vi "Main.vi"() -> ()   [LabVIEW 2011]
uses:
  granula_llb.lvlib
panel:
  out "tdms path":string caption="ЗАДАНИЕ, мин"
  in  "Участок 2 выключить":bool
  out "Проведение второго участка":bool
  in  "участок 2 включить":bool
  in  "Cal v 2":i16
  in  "S2 t 2":i16
  in  "S2v 2":i16
  in  "S1 t 2":i16
  in  "S1 v 2":i16
  in  "МАКРО СТОП":bool
  in  "НАГРЕВ НАЧАТЬ АВТО":bool
  in  "ВЫГРУЗИТЬ":bool
  in  "ЗАГРУЗИТЬ":bool
  out "T7":string caption="Т7"
  in  "Cal v":i16
  in  "S2 t":i16
  in  "S2v":i16
  in  "S1 t":i16
  in  "S1 v":i16
  in  "A":i16
  in  "Hz":i16
  in  "T7":i16
  in  "T6":i16
  in  "T5":i16
  in  "T4":i16
  in  "T3":i16
  in  "T2":i16
  in  "T1":i16
  in  "error":i16
  out "Нагрев включен":bool caption="Нагрев"
  out "Готовность привода":bool caption="Готов"
  out "Авария привода":bool caption="Авария"
  in  "Y20-Y57":i32
  in  "X100-X137":i32
  in  "X40-X77":i32
  out "Команда выход":bool caption="ОТКРЫТ"
  in  "Закалка выкл":bool
  in  "Закалка вкл":bool
  in  "Телегу в точку А":bool
  in  "Телегу под печь":bool
  in  "Телегу на разгрузку":bool
  in  "Под закрыть":bool
  in  "ПОД открыnnть":bool
  in  "Цепи вниз":bool
  in  "Цепи наверх":bool
  in  "Домкрат вверх":bool
  in  "Домкрат вниз":bool
  out "Закалка":bool
  out "Участок 2":bool
  out "Участок 1":bool
  out "АВТО ЦИКЛ":bool
  out "текущее время":string
  in  "Цикл пуск":bool
  in  "Цикл стоп":bool
  in  "Просмотр графика":bool
  in  "Наладка":bool
  in  "ВЫХОД":bool
  out "УПРАВЛЕНИЕ С PLC":bool
  out "ВОДА":bool
  out "ВОДА 2":bool
  out "ВОДА 3":bool
  out "ВОДА 4":bool
  out "Проведение закалки":bool
  out "Зак зад":string caption="ЗАДАНИЕ, мин"
  out "Зак выд":string caption="ВЫДЕРЖКА, мин"
  out "Уч2 Тзад":string caption="ЗАДАНИЕ, град"
  out "Уч2 Т":string caption="ТЕМПЕРАТУРА, град"
  out "Уч2 Выд зад":string caption="ЗАДАНИЕ, мин"
  out "Уч2 Выд":string caption="ВЫДЕРЖКА, мин"
  out "Уч1 Т зад":string caption="ЗАДАНИЕ, град"
  out "Уч1 Т":string caption="ТЕМПЕРАТУРА, град"
  out "Уч1 выд зад":string caption="ЗАДАНИЕ, мин"
  out "Уч1 Выд":string caption="ВЫДЕРЖКА, мин"
  out "ПОД ЗАКРЫТ":bool caption="ЗАКРЫТ"
  out "ПОД ОТКРЫТ":bool caption="ОТКРЫТ"
  out "Двиг Ток А":string caption="ТОК А"
  out "Двиг част Hz":string caption="ЧАСТОТА Hz"
  out "T5":string caption="Т5"
  out "T6":string caption="Т6"
  out "T3":string caption="Т3"
  out "T4":string caption="Т4"
  out "T1":string caption="Т1"
  out "T2":string caption="Т2"
  out "ТОЧКА А":bool
  out "ЗАЦЕП":bool
  out "РАЗГРУЗКА":bool
  out "Цепи внизу":bool caption="Закал"
  out "Цепи среднее":bool caption="Зацеп"
  out "Цепи вверху":bool caption="Камера"
  out "Домкрат внизу":bool caption="Закал"
  out "Домкрат вверху":bool caption="Зацеп"
  # "КАМЕРА НАГРЕВА"
  # "НАГРЕВ"
  # "МАКРО"
  # "ПОД"
  # "ЦЕПИ"
  # "Д\nО\nМ\nК\nР\nА\nТ"
  # "Д\nО\nМ\nК\nР\nА\nТ"
  # "САДКА"
  # "Т\nЕ\nЛ\nЕ\nГ\nА"
  # "САДКА"
  # "ИНДИКАЦИЯ ПРОТОКА ВОДЫ"
  # "СТУПЕНЬ №2"
  # "СТУПЕНЬ №1"
  # "ЗАКАЛКА"
  # "ПРОВЕДЕНИЕ ЗАКАЛКИ"
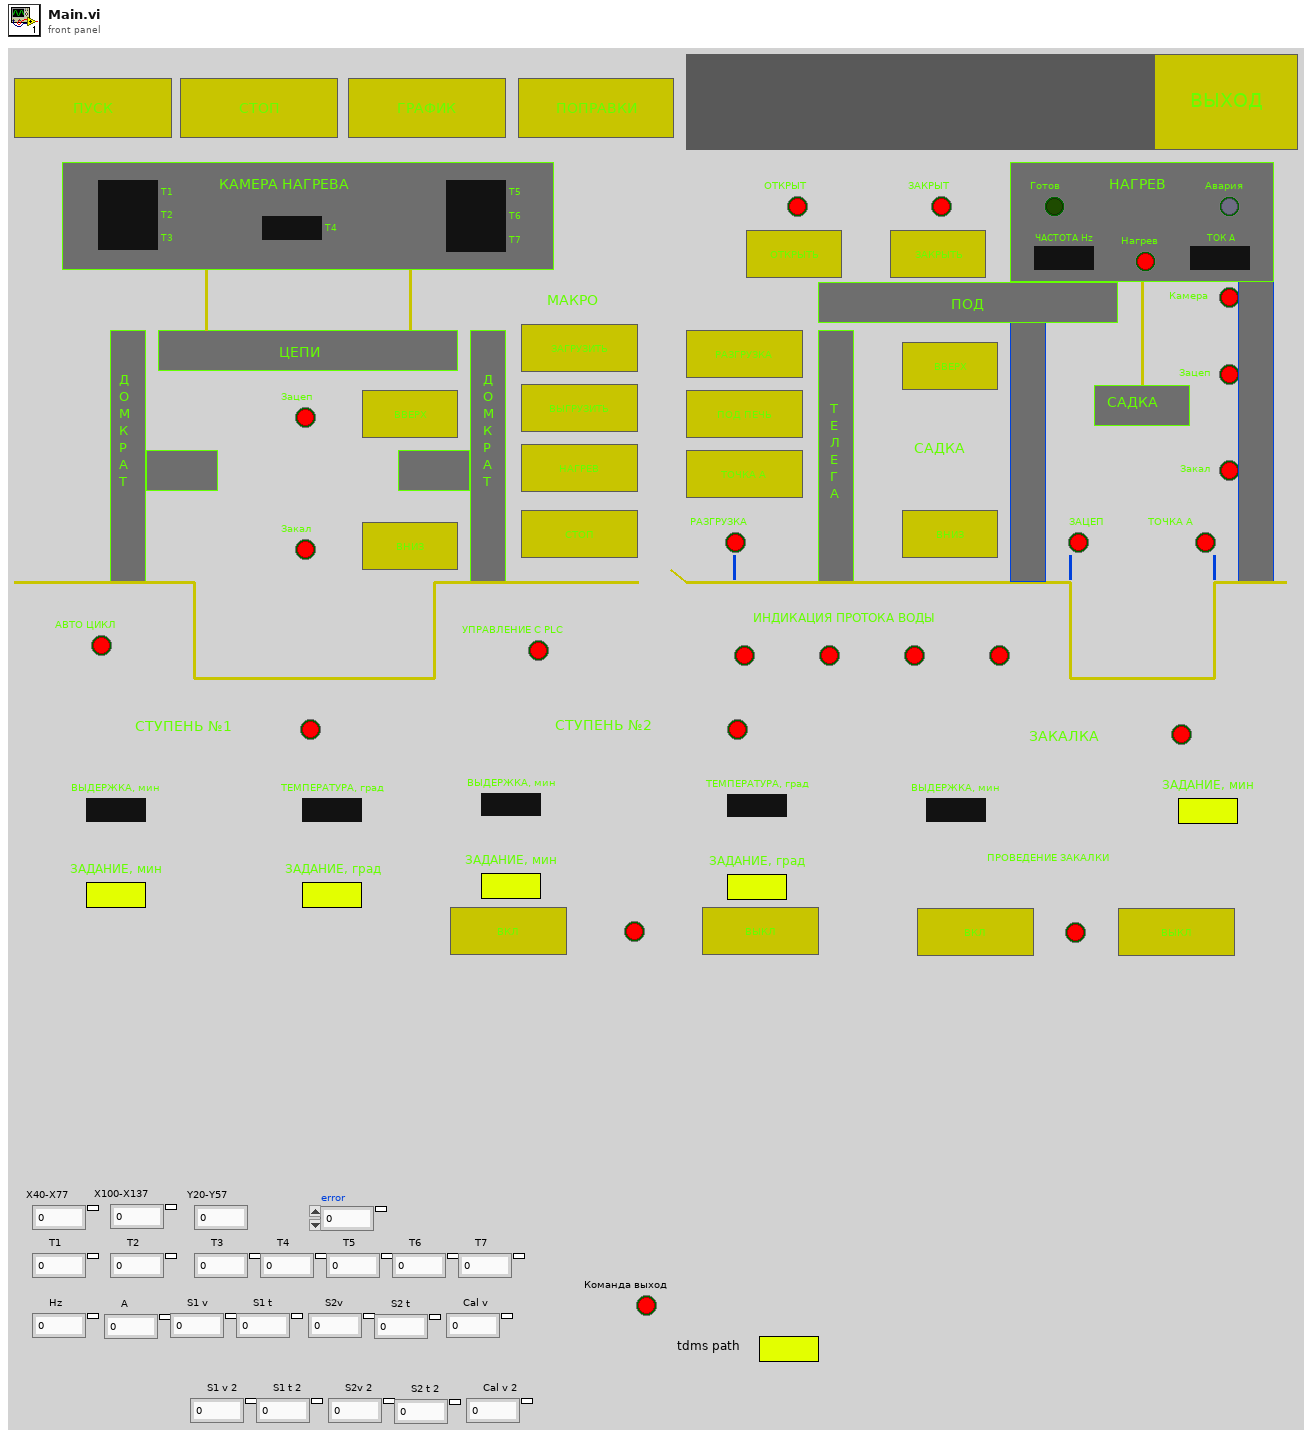
[diagram p1: front panel]
types:
  T1 = enum16{"big-endian, network order", "native, host order", "little-endian"}
  T2 = enum16{"open", "open or create", "create or replace", "create", "open (read-only)"}
  T3 = enum16{"open", "replace", "create", "open or create", "replace or create", "replace or create with confirmation"}
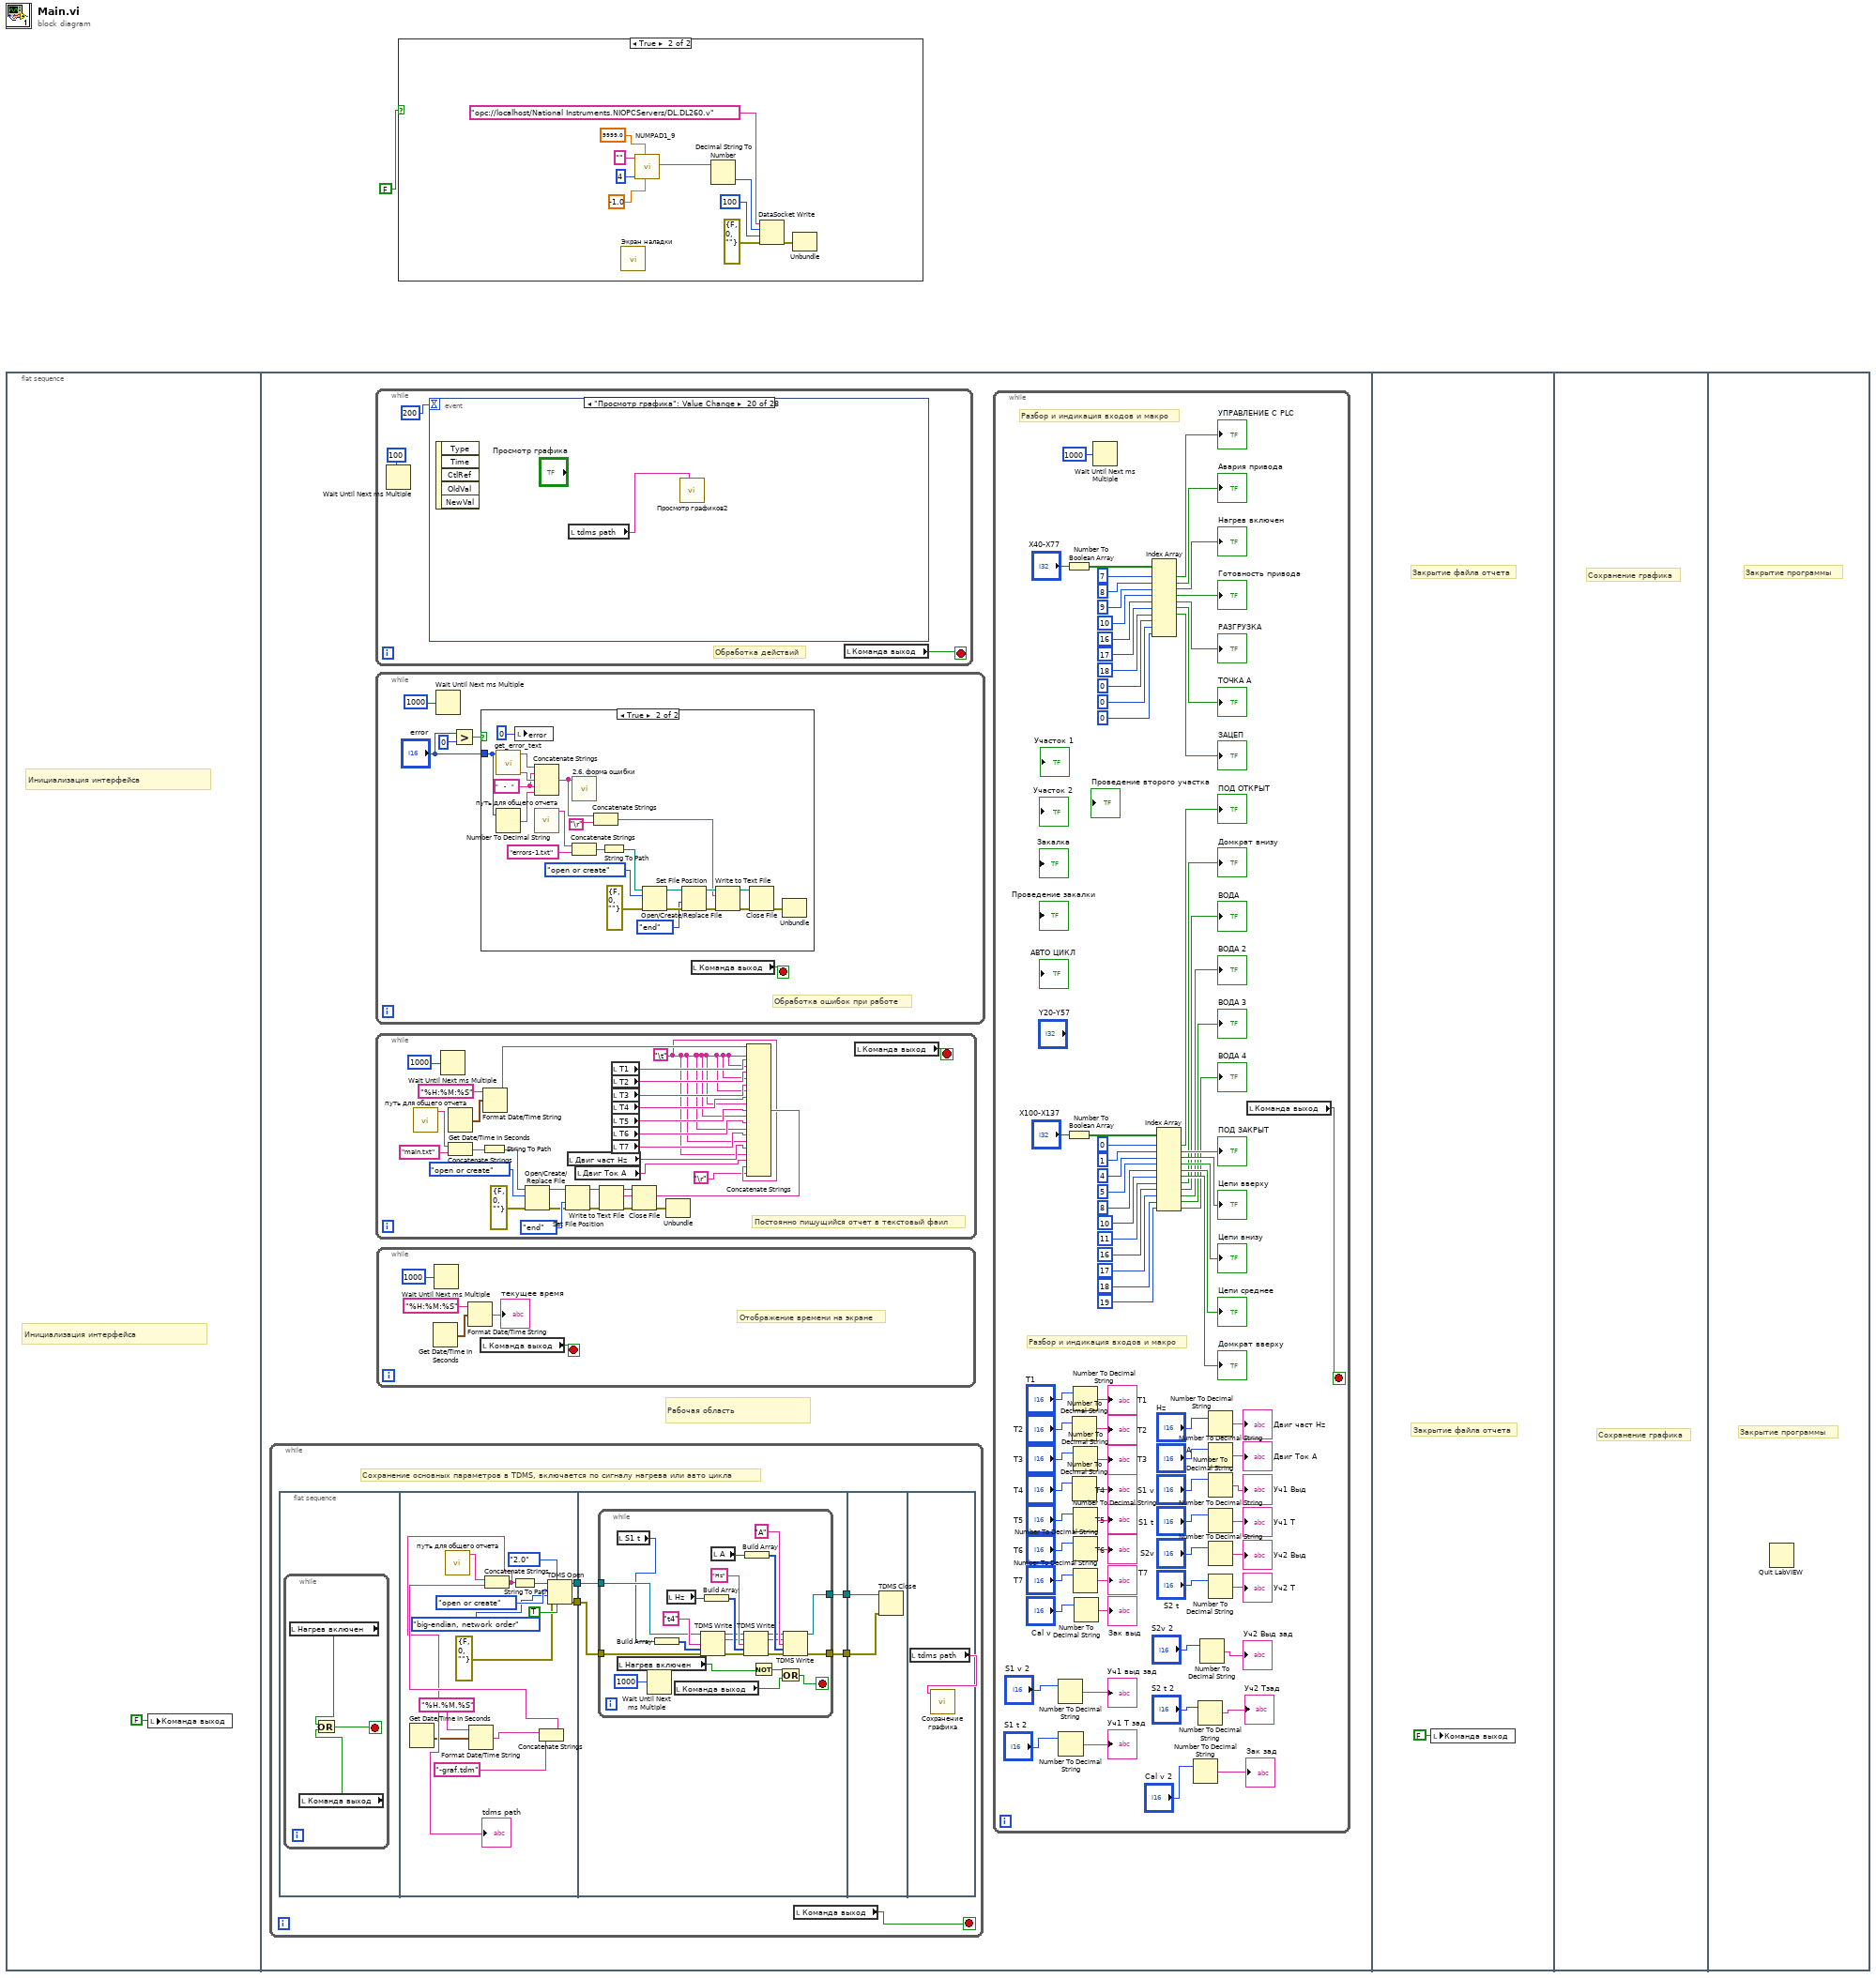
[diagram p0: block diagram]
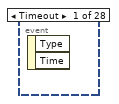
[diagram p3: hidden frame]
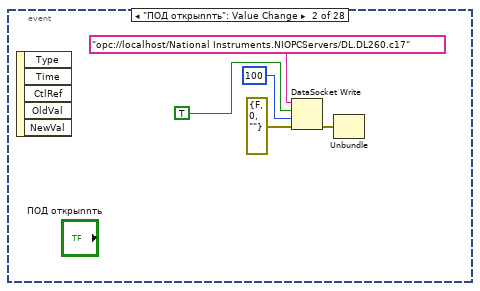
[diagram p4: hidden frame]
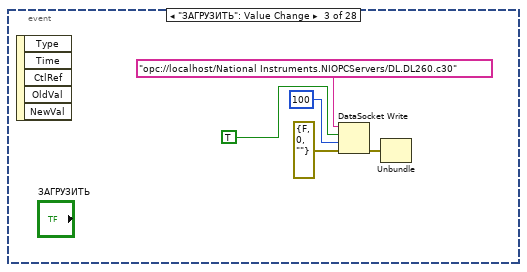
[diagram p5: hidden frame]
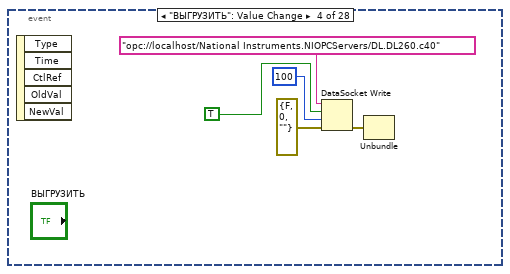
[diagram p6: hidden frame]
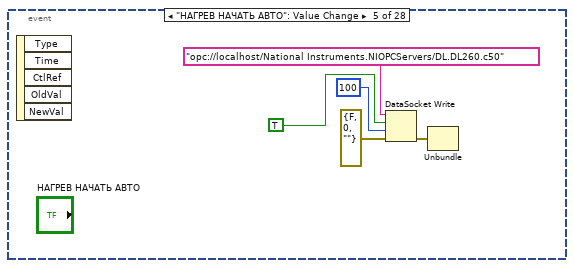
[diagram p7: hidden frame]
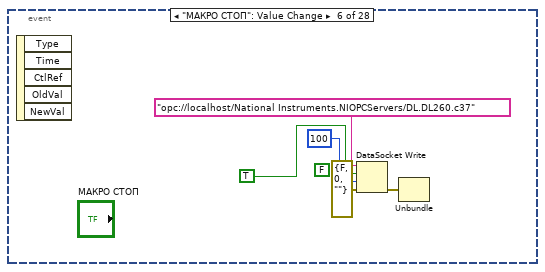
[diagram p8: hidden frame]
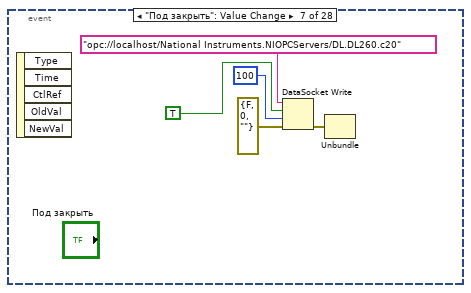
[diagram p9: hidden frame]
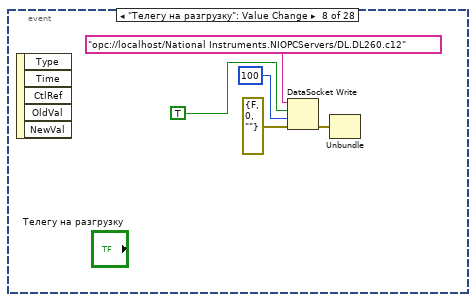
[diagram p10: hidden frame]
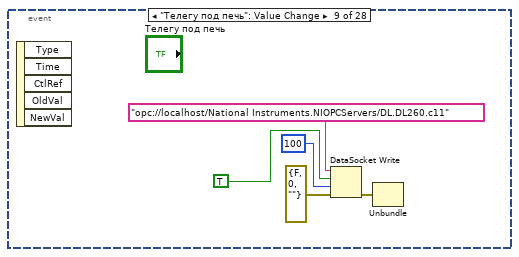
[diagram p11: hidden frame]
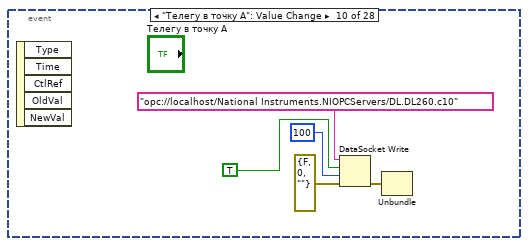
[diagram p12: hidden frame]
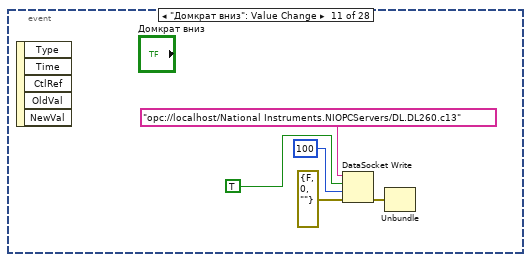
[diagram p13: hidden frame]
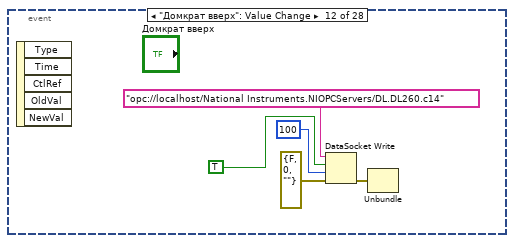
[diagram p14: hidden frame]
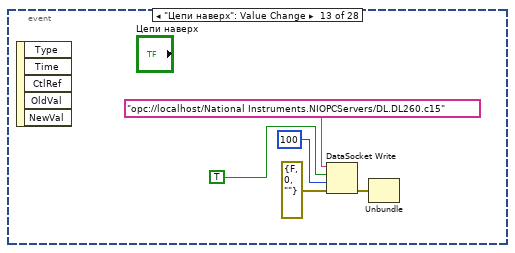
[diagram p15: hidden frame]
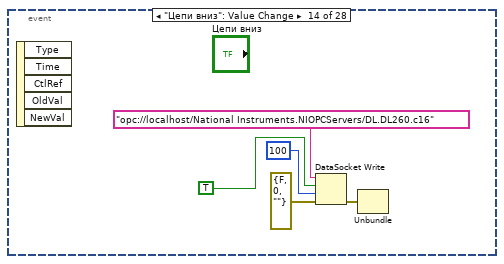
[diagram p16: hidden frame]
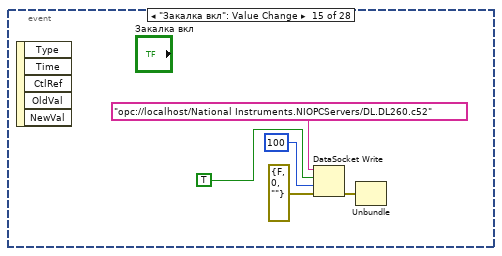
[diagram p17: hidden frame]
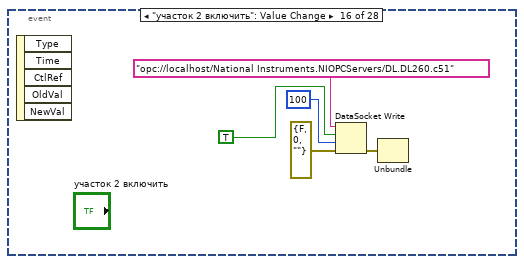
[diagram p18: hidden frame]
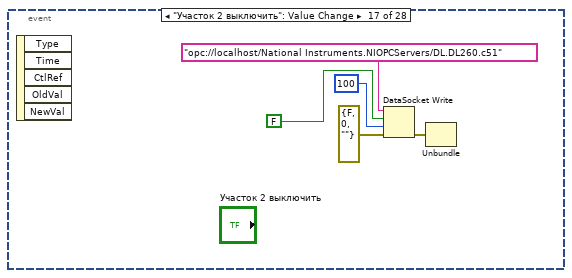
[diagram p19: hidden frame]
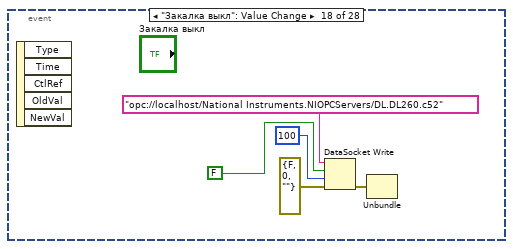
[diagram p20: hidden frame]
diagram:
  n1 = flat-sequence {
    frame #0 {
      # "Инициализация интерфейса"
      # "Инициализация интерфейса"
      n2 = local write "Команда выход"(FALSE ("Команда выход")) -> ()
    }
    frame #1 {
      # "Рабочая область"
      n3 = while {
        stop <- w3 stop-if-true
        # "Сохранение основных параметров в TDMS, включается по сигналу нагрева или авто цикла"
        n4 = flat-sequence {
          tunnel: [w16] -> w7
          tunnel: [w15] -> w6
          tunnel: w7 -> [w29]
          tunnel: w6 -> [w28]
          tunnel: [w27] -> w5
          tunnel: [w26] -> w4
          tunnel: w5 -> [w55]
          tunnel: w4 -> [w54]
          frame #0 {
            n5 = while {
              stop <- w10 stop-if-true
              n6 = local read "Нагрев включен"() -> (w8:bool)
              n7 = local read "Команда выход"() -> (w9:bool)
              n8 = Or(x=w8, y=w9) -> (x .or. y?=w10:bool)
            }
          }
          frame #1 {
            n9 = Get Date/Time In Seconds() -> (seconds since 1Jan1904=w11:timestamp)
            n10 = call "путь для общего отчета.vi"() -> ("path_out 2"=w25:string)  [unwired: 11 in]
            n11 = Format Date/Time String(time format string (%c)="%H.%M.%S", seconds (now)=w11) -> (date/time string=w13:string)  [unwired: 1 in]
            n12 = Concatenate Strings(w13, "-graf.tdm") -> (w17:string)
            n13 = Concatenate Strings(w25, w17) -> (w14:string)
            "tdms path" <- w14
            n14 = String To Path(string=w14) -> (path=w24:path)
            n15 = TDMS Open(6:TRUE ("disable buffering? (T)"), 7:enum16{"1.0", "2.0"}."2.0" ("file format version (2.0)"), 8:errorcluster {"status"=FALSE, "code"=0, "source"=""} ("error in (no error)"), 9:T1."big-endian, network order" ("byte order (2:little-endian)"), 10:T2."open or create" ("operation (0:open)"), 11:w24) -> (0:w15:errorcluster, 3:w16:refnum<k34>)
          }
          frame #2 {
            n16 = while {
              tunnel: w29 -> [w38]
              tunnel: w28 -> [w37]
              tunnel: [w36] -> w27
              tunnel: [w35] -> w26
              stop <- w32 stop-if-true
              n17 = local read "S1 t"() -> (w30:i16)
              n18 = local read "Нагрев включен"() -> (w31:bool)
              n19 = Wait Until Next ms Multiple(millisecond multiple=u32 1000) -> ()  [unwired: 1 out]
              n20 = Build Array(w30) -> (w53:i16[])
              n21 = local read "Hz"() -> (w44:i16)
              n22 = local read "Команда выход"() -> (w33:bool)
              n23 = TDMS Write(0:w38, 7:"t4", 9:w53, 11:w37) -> (4:w42:refnum<k34>, 6:w41:string, 15:w40:errorcluster)  [unwired: 2 in, 1 out]
              n24 = Build Array(w44) -> (w50:i16[])
              n25 = local read "A"() -> (w45:i16)
              n26 = TDMS Write(0:w42, 5:w41, 7:"Hz", 9:w50, 11:w40) -> (4:w47:refnum<k34>, 6:w43:string, 15:w46:errorcluster)  [unwired: 1 in, 1 out]
              n27 = Build Array(w45) -> (w48:i16[])
              n28 = Not(x=w31) -> (.not. x?=w34:bool)
              n29 = Or(x=w34, y=w33) -> (x .or. y?=w32:bool)
              n30 = TDMS Write(0:w47, 5:w43, 7:"A", 9:w48, 11:w46) -> (4:w36:refnum<k34>, 15:w35:errorcluster)  [unwired: 1 in, 2 out]
            }
          }
          frame #3 {
            n31 = TDMS Close(8:w54, 11:w55) -> ()  [unwired: 2 out]
          }
          frame #4 {
            n32 = local read "tdms path"() -> (w56:string)
            n33 = call "Сохранение графика.vi"("String"=w56) -> ()  [unwired: 11 in]
          }
        }
        n34 = local read "Команда выход"() -> (w3:bool)
      }
      n35 = while {
        stop <- w62 stop-if-true
        # "Обработка действий"
        n36 = Wait Until Next ms Multiple(millisecond multiple=u32 100) -> ()  [unwired: 1 out]
        n37 = event shown="[19] \"Просмотр графика\": Value Change" {
          selector: _ -> [_ _ _ _ _ _ _ _ _ _ _ _ _ _ _ _ _ _ _ _ _ _ _ _ _ _ _ _]
          dyn-events: _ -> [_ _ _ _ _ _ _ _ _ _ _ _ _ _ _ _ _ _ _ _ _ _ _ _ _ _ _ _]
          timeout: 200 -> [_ _ _ _ _ _ _ _ _ _ _ _ _ _ _ _ _ _ _ _ _ _ _ _ _ _ _ _]
          event Timeout {
            n38 = event-data() -> ()  [unwired: 1 in, 2 out]
          }
          event "ПОД открыnnть": Value Change {
            n39 = event-data() -> ()  [unwired: 1 in, 5 out]
            n40 = DataSocket Write(8:errorcluster {"status"=FALSE, "code"=0, "source"=""} ("error in (no error)"), 9:100 ("ms timeout (0)"), 10:TRUE, 11:"opc://localhost/National Instruments.NIOPCServers/DL.DL260.c17" ("connection in")) -> (0:w69:errorcluster)  [unwired: 2 out]
            n41 = Unbundle(w69) -> ()  [unwired: 3 out]
          }
          event "ЗАГРУЗИТЬ": Value Change {
            n42 = event-data() -> ()  [unwired: 1 in, 5 out]
            n43 = DataSocket Write(8:errorcluster {"status"=FALSE, "code"=0, "source"=""} ("error in (no error)"), 9:100 ("ms timeout (0)"), 10:TRUE, 11:"opc://localhost/National Instruments.NIOPCServers/DL.DL260.c30" ("connection in")) -> (0:w74:errorcluster)  [unwired: 2 out]
            n44 = Unbundle(w74) -> ()  [unwired: 3 out]
          }
          event "ВЫГРУЗИТЬ": Value Change {
            n45 = event-data() -> ()  [unwired: 1 in, 5 out]
            n46 = DataSocket Write(8:errorcluster {"status"=FALSE, "code"=0, "source"=""} ("error in (no error)"), 9:100 ("ms timeout (0)"), 10:TRUE, 11:"opc://localhost/National Instruments.NIOPCServers/DL.DL260.c40" ("connection in")) -> (0:w79:errorcluster)  [unwired: 2 out]
            n47 = Unbundle(w79) -> ()  [unwired: 3 out]
          }
          event "НАГРЕВ НАЧАТЬ АВТО": Value Change {
            n48 = event-data() -> ()  [unwired: 1 in, 5 out]
            n49 = DataSocket Write(8:errorcluster {"status"=FALSE, "code"=0, "source"=""} ("error in (no error)"), 9:100 ("ms timeout (0)"), 10:TRUE, 11:"opc://localhost/National Instruments.NIOPCServers/DL.DL260.c50" ("connection in")) -> (0:w84:errorcluster)  [unwired: 2 out]
            n50 = Unbundle(w84) -> ()  [unwired: 3 out]
          }
          event "МАКРО СТОП": Value Change {
            (unwired) FALSE ("status")
            n51 = event-data() -> ()  [unwired: 1 in, 5 out]
            n52 = DataSocket Write(8:errorcluster {"status"=FALSE, "code"=0, "source"=""} ("error in (no error)"), 9:100 ("ms timeout (0)"), 10:TRUE, 11:"opc://localhost/National Instruments.NIOPCServers/DL.DL260.c37" ("connection in")) -> (0:w89:errorcluster)  [unwired: 2 out]
            n53 = Unbundle(w89) -> ()  [unwired: 3 out]
          }
          event "Под закрыть": Value Change {
            n54 = event-data() -> ()  [unwired: 1 in, 5 out]
            n55 = DataSocket Write(8:errorcluster {"status"=FALSE, "code"=0, "source"=""} ("error in (no error)"), 9:100 ("ms timeout (0)"), 10:TRUE, 11:"opc://localhost/National Instruments.NIOPCServers/DL.DL260.c20" ("connection in")) -> (0:w94:errorcluster)  [unwired: 2 out]
            n56 = Unbundle(w94) -> ()  [unwired: 3 out]
          }
          event "Телегу на разгрузку": Value Change {
            n57 = event-data() -> ()  [unwired: 1 in, 5 out]
            n58 = DataSocket Write(8:errorcluster {"status"=FALSE, "code"=0, "source"=""} ("error in (no error)"), 9:100 ("ms timeout (0)"), 10:TRUE, 11:"opc://localhost/National Instruments.NIOPCServers/DL.DL260.c12" ("connection in")) -> (0:w99:errorcluster)  [unwired: 2 out]
            n59 = Unbundle(w99) -> ()  [unwired: 3 out]
          }
          event "Телегу под печь": Value Change {
            n60 = event-data() -> ()  [unwired: 1 in, 5 out]
            n61 = DataSocket Write(8:errorcluster {"status"=FALSE, "code"=0, "source"=""} ("error in (no error)"), 9:100 ("ms timeout (0)"), 10:TRUE, 11:"opc://localhost/National Instruments.NIOPCServers/DL.DL260.c11" ("connection in")) -> (0:w104:errorcluster)  [unwired: 2 out]
            n62 = Unbundle(w104) -> ()  [unwired: 3 out]
          }
          event "Телегу в точку А": Value Change {
            n63 = event-data() -> ()  [unwired: 1 in, 5 out]
            n64 = DataSocket Write(8:errorcluster {"status"=FALSE, "code"=0, "source"=""} ("error in (no error)"), 9:100 ("ms timeout (0)"), 10:TRUE, 11:"opc://localhost/National Instruments.NIOPCServers/DL.DL260.c10" ("connection in")) -> (0:w109:errorcluster)  [unwired: 2 out]
            n65 = Unbundle(w109) -> ()  [unwired: 3 out]
          }
          event "Домкрат вниз": Value Change {
            n66 = event-data() -> ()  [unwired: 1 in, 5 out]
            n67 = DataSocket Write(8:errorcluster {"status"=FALSE, "code"=0, "source"=""} ("error in (no error)"), 9:100 ("ms timeout (0)"), 10:TRUE, 11:"opc://localhost/National Instruments.NIOPCServers/DL.DL260.c13" ("connection in")) -> (0:w114:errorcluster)  [unwired: 2 out]
            n68 = Unbundle(w114) -> ()  [unwired: 3 out]
          }
          event "Домкрат вверх": Value Change {
            n69 = event-data() -> ()  [unwired: 1 in, 5 out]
            n70 = DataSocket Write(8:errorcluster {"status"=FALSE, "code"=0, "source"=""} ("error in (no error)"), 9:100 ("ms timeout (0)"), 10:TRUE, 11:"opc://localhost/National Instruments.NIOPCServers/DL.DL260.c14" ("connection in")) -> (0:w119:errorcluster)  [unwired: 2 out]
            n71 = Unbundle(w119) -> ()  [unwired: 3 out]
          }
          event "Цепи наверх": Value Change {
            n72 = event-data() -> ()  [unwired: 1 in, 5 out]
            n73 = DataSocket Write(8:errorcluster {"status"=FALSE, "code"=0, "source"=""} ("error in (no error)"), 9:100 ("ms timeout (0)"), 10:TRUE, 11:"opc://localhost/National Instruments.NIOPCServers/DL.DL260.c15" ("connection in")) -> (0:w124:errorcluster)  [unwired: 2 out]
            n74 = Unbundle(w124) -> ()  [unwired: 3 out]
          }
          event "Цепи вниз": Value Change {
            n75 = event-data() -> ()  [unwired: 1 in, 5 out]
            n76 = DataSocket Write(8:errorcluster {"status"=FALSE, "code"=0, "source"=""} ("error in (no error)"), 9:100 ("ms timeout (0)"), 10:TRUE, 11:"opc://localhost/National Instruments.NIOPCServers/DL.DL260.c16" ("connection in")) -> (0:w129:errorcluster)  [unwired: 2 out]
            n77 = Unbundle(w129) -> ()  [unwired: 3 out]
          }
          event "Закалка вкл": Value Change {
            n78 = event-data() -> ()  [unwired: 1 in, 5 out]
            n79 = DataSocket Write(8:errorcluster {"status"=FALSE, "code"=0, "source"=""} ("error in (no error)"), 9:100 ("ms timeout (0)"), 10:TRUE, 11:"opc://localhost/National Instruments.NIOPCServers/DL.DL260.c52" ("connection in")) -> (0:w134:errorcluster)  [unwired: 2 out]
            n80 = Unbundle(w134) -> ()  [unwired: 3 out]
          }
          event "участок 2 включить": Value Change {
            n81 = event-data() -> ()  [unwired: 1 in, 5 out]
            n82 = DataSocket Write(8:errorcluster {"status"=FALSE, "code"=0, "source"=""} ("error in (no error)"), 9:100 ("ms timeout (0)"), 10:TRUE, 11:"opc://localhost/National Instruments.NIOPCServers/DL.DL260.c51" ("connection in")) -> (0:w139:errorcluster)  [unwired: 2 out]
            n83 = Unbundle(w139) -> ()  [unwired: 3 out]
          }
          event "Участок 2 выключить": Value Change {
            n84 = event-data() -> ()  [unwired: 1 in, 5 out]
            n85 = DataSocket Write(8:errorcluster {"status"=FALSE, "code"=0, "source"=""} ("error in (no error)"), 9:100 ("ms timeout (0)"), 10:FALSE, 11:"opc://localhost/National Instruments.NIOPCServers/DL.DL260.c51" ("connection in")) -> (0:w144:errorcluster)  [unwired: 2 out]
            n86 = Unbundle(w144) -> ()  [unwired: 3 out]
          }
          event "Закалка выкл": Value Change {
            n87 = event-data() -> ()  [unwired: 1 in, 5 out]
            n88 = DataSocket Write(8:errorcluster {"status"=FALSE, "code"=0, "source"=""} ("error in (no error)"), 9:100 ("ms timeout (0)"), 10:FALSE, 11:"opc://localhost/National Instruments.NIOPCServers/DL.DL260.c52" ("connection in")) -> (0:w149:errorcluster)  [unwired: 2 out]
            n89 = Unbundle(w149) -> ()  [unwired: 3 out]
          }
          event "Наладка": Value Change {
            n90 = event-data() -> ()  [unwired: 1 in, 5 out]
            n91 = call "Корректировка.vi"() -> ()  [unwired: 12 in]
          }
          event "Просмотр графика": Value Change {
            n92 = event-data() -> ()  [unwired: 1 in, 5 out]
            n93 = local read "tdms path"() -> (w150:string)
            n94 = call "Просмотр графиков2.vi"("tdm"=w150) -> ()  [unwired: 11 in]
          }
          event "Цикл пуск": Value Change {
            n95 = event-data() -> ()  [unwired: 1 in, 5 out]
            n96 = DataSocket Write(8:errorcluster {"status"=FALSE, "code"=0, "source"=""} ("error in (no error)"), 9:100 ("ms timeout (0)"), 10:TRUE, 11:"opc://localhost/National Instruments.NIOPCServers/DL.DL260.c50" ("connection in")) -> (0:w155:errorcluster)  [unwired: 2 out]
            n97 = Unbundle(w155) -> ()  [unwired: 3 out]
          }
          event "Цикл стоп": Value Change {
            n98 = event-data() -> ()  [unwired: 1 in, 5 out]
            n99 = DataSocket Write(8:errorcluster {"status"=FALSE, "code"=0, "source"=""} ("error in (no error)"), 9:100 ("ms timeout (0)"), 10:FALSE, 11:"opc://localhost/National Instruments.NIOPCServers/DL.DL260.c50" ("connection in")) -> (0:w160:errorcluster)  [unwired: 2 out]
            n100 = Unbundle(w160) -> ()  [unwired: 3 out]
          }
          event "Уч1 выд зад": Mouse Down {
            n101 = event-data() -> ()  [unwired: 1 in, 7 out]
            n102 = local read "Уч1 выд зад"() -> (w161:string)
            n103 = call "NUMPAD1_9.vi"("МИНИМАЛЬНОЕ ЗНАЧЕНИЕ"=-1.0, "МАКСИМАЛЬНОЕ ЗНАЧЕНИЕ"=9999.0, "ДЛИННА СЛОВА"=i8 4, "ТЕКУЩЕЕ ЗНАЧЕНИЕ"=w161) -> ("НОВОЕ ЗНАЧЕНИЕ"=w166:string)  [unwired: 7 in]
            n104 = Decimal String To Number(string=w166) -> (number=w162:i32)  [unwired: 2 in, 1 out]
            n105 = DataSocket Write(8:errorcluster {"status"=FALSE, "code"=0, "source"=""} ("error in (no error)"), 9:100 ("ms timeout (0)"), 10:w162, 11:"opc://localhost/National Instruments.NIOPCServers/DL.DL260.v700" ("connection in")) -> (0:w170:errorcluster)  [unwired: 2 out]
            n106 = Unbundle(w170) -> ()  [unwired: 3 out]
          }
          event "Уч1 Т зад": Mouse Down {
            n107 = event-data() -> ()  [unwired: 1 in, 7 out]
            n108 = local read "Уч1 Т зад"() -> (w171:string)
            n109 = call "NUMPAD1_9.vi"("МИНИМАЛЬНОЕ ЗНАЧЕНИЕ"=-1.0, "МАКСИМАЛЬНОЕ ЗНАЧЕНИЕ"=9999.0, "ДЛИННА СЛОВА"=i8 4, "ТЕКУЩЕЕ ЗНАЧЕНИЕ"=w171) -> ("НОВОЕ ЗНАЧЕНИЕ"=w176:string)  [unwired: 7 in]
            n110 = Decimal String To Number(string=w176) -> (number=w172:i32)  [unwired: 2 in, 1 out]
            n111 = DataSocket Write(8:errorcluster {"status"=FALSE, "code"=0, "source"=""} ("error in (no error)"), 9:100 ("ms timeout (0)"), 10:w172, 11:"opc://localhost/National Instruments.NIOPCServers/DL.DL260.v701" ("connection in")) -> (0:w180:errorcluster)  [unwired: 2 out]
            n112 = Unbundle(w180) -> ()  [unwired: 3 out]
          }
          event "Уч2 Выд зад": Mouse Down {
            n113 = event-data() -> ()  [unwired: 1 in, 7 out]
            n114 = local read "Уч2 Выд зад"() -> (w181:string)
            n115 = call "NUMPAD1_9.vi"("МИНИМАЛЬНОЕ ЗНАЧЕНИЕ"=-1.0, "МАКСИМАЛЬНОЕ ЗНАЧЕНИЕ"=9999.0, "ДЛИННА СЛОВА"=i8 4, "ТЕКУЩЕЕ ЗНАЧЕНИЕ"=w181) -> ("НОВОЕ ЗНАЧЕНИЕ"=w186:string)  [unwired: 7 in]
            n116 = Decimal String To Number(string=w186) -> (number=w182:i32)  [unwired: 2 in, 1 out]
            n117 = DataSocket Write(8:errorcluster {"status"=FALSE, "code"=0, "source"=""} ("error in (no error)"), 9:100 ("ms timeout (0)"), 10:w182, 11:"opc://localhost/National Instruments.NIOPCServers/DL.DL260.v710" ("connection in")) -> (0:w190:errorcluster)  [unwired: 2 out]
            n118 = Unbundle(w190) -> ()  [unwired: 3 out]
          }
          event "Уч2 Тзад": Mouse Down {
            n119 = event-data() -> ()  [unwired: 1 in, 7 out]
            n120 = local read "Уч2 Тзад"() -> (w191:string)
            n121 = call "NUMPAD1_9.vi"("МИНИМАЛЬНОЕ ЗНАЧЕНИЕ"=-1.0, "МАКСИМАЛЬНОЕ ЗНАЧЕНИЕ"=9999.0, "ДЛИННА СЛОВА"=i8 4, "ТЕКУЩЕЕ ЗНАЧЕНИЕ"=w191) -> ("НОВОЕ ЗНАЧЕНИЕ"=w196:string)  [unwired: 7 in]
            n122 = Decimal String To Number(string=w196) -> (number=w192:i32)  [unwired: 2 in, 1 out]
            n123 = DataSocket Write(8:errorcluster {"status"=FALSE, "code"=0, "source"=""} ("error in (no error)"), 9:100 ("ms timeout (0)"), 10:w192, 11:"opc://localhost/National Instruments.NIOPCServers/DL.DL260.v711" ("connection in")) -> (0:w200:errorcluster)  [unwired: 2 out]
            n124 = Unbundle(w200) -> ()  [unwired: 3 out]
          }
          event "Зак зад": Mouse Down {
            n125 = event-data() -> ()  [unwired: 1 in, 7 out]
            n126 = local read "Зак зад"() -> (w201:string)
            n127 = call "NUMPAD1_9.vi"("МИНИМАЛЬНОЕ ЗНАЧЕНИЕ"=-1.0, "МАКСИМАЛЬНОЕ ЗНАЧЕНИЕ"=9999.0, "ДЛИННА СЛОВА"=i8 4, "ТЕКУЩЕЕ ЗНАЧЕНИЕ"=w201) -> ("НОВОЕ ЗНАЧЕНИЕ"=w206:string)  [unwired: 7 in]
            n128 = Decimal String To Number(string=w206) -> (number=w202:i32)  [unwired: 2 in, 1 out]
            n129 = DataSocket Write(8:errorcluster {"status"=FALSE, "code"=0, "source"=""} ("error in (no error)"), 9:100 ("ms timeout (0)"), 10:w202, 11:"opc://localhost/National Instruments.NIOPCServers/DL.DL260.v720" ("connection in")) -> (0:w210:errorcluster)  [unwired: 2 out]
            n130 = Unbundle(w210) -> ()  [unwired: 3 out]
          }
          event "ВЫХОД": Value Change {
            n131 = event-data() -> ()  [unwired: 1 in, 5 out]
            "Команда выход" <- TRUE ("Команда выход")
          }
        }
        n132 = local read "Команда выход"() -> (w62:bool)
      }
      n133 = while {
        stop <- w212 stop-if-true
        # "Обработка ошибок при работе"
        n134 = Wait Until Next ms Multiple(millisecond multiple=u32 1000) -> ()  [unwired: 1 out]
        n135 = Greater?(x="error", y=i16 0) -> (0:w215:bool)
        n136 = case shown="True" w215 {
          tunnel: "error" -> [_ w217]
          frame False {
          }
          frame True {
            w219 = "   -   " ("string")
            n137 = call "get_error_text.vi"("Код ошибки"=w217) -> ("Событие"=w221:string, "Механизм"=w222:string)  [unwired: 9 in]
            n138 = Number To Decimal String(number=w217) -> (decimal integer string=w218:string)  [unwired: 1 in]
            n139 = local write "error"(i16 0 ("Ошибка1")) -> ()
            n140 = Concatenate Strings(w222, w219, w221, w219, w218) -> (w223:string)
            n141 = call "путь для общего отчета.vi"() -> ("path_out 2"=w224:string)  [unwired: 11 in]
            n142 = call "2.6. форма ошибки.vi"("Описание ошибки"=w223) -> ()  [unwired: 11 in]
            n143 = Concatenate Strings(w224, "errors-1.txt") -> (w237:string)
            n144 = Concatenate Strings(w223, "\r") -> (w225:string)
            n145 = String To Path(string=w237) -> (path=w239:path)
            n146 = Open/Create/Replace File(file path (use dialog)=w239, error in=errorcluster {"status"=FALSE, "code"=0, "source"=""}, operation (0:open)=T3."open or create") -> (refnum out=w232:refnum<file>, error out=w234:errorcluster)  [unwired: 3 in, 1 out]
            n147 = Set File Position(refnum=w232, from (0:start)=enum16{"start", "end", "current"}."end", error in=w234) -> (refnum out=w230:refnum<file>, error out=w231:errorcluster)  [unwired: 1 in]
            n148 = Write to Text File(file (use dialog)=w230, text=w225, error in=w231) -> (refnum out=w229:refnum<file>, error out=w228:errorcluster)  [unwired: 1 in, 1 out]
            n149 = Close File(refnum=w229, error in=w228) -> (error out=w227:errorcluster)  [unwired: 1 out]
            n150 = Unbundle(w227) -> ()  [unwired: 3 out]
          }
        }
        n151 = local read "Команда выход"() -> (w212:bool)
      }
      n152 = while {
        stop <- w251 stop-if-true
        w241 = "\t"
        # "Постоянно пишущийся отчет в текстовый фаил"
        n153 = call "путь для общего отчета.vi"() -> ("path_out 2"=w253:string)  [unwired: 11 in]
        n154 = Wait Until Next ms Multiple(millisecond multiple=u32 1000) -> ()  [unwired: 1 out]
        n155 = Get Date/Time In Seconds() -> (seconds since 1Jan1904=w256:timestamp)
        n156 = Concatenate Strings(w253, "main.txt") -> (w259:string)
        n157 = String To Path(string=w259) -> (path=w257:path)
        n158 = Format Date/Time String(time format string (%c)="%H:%M:%S", seconds (now)=w256) -> (date/time string=w252:string)  [unwired: 1 in]
        n159 = Open/Create/Replace File(file path (use dialog)=w257, error in=errorcluster {"status"=FALSE, "code"=0, "source"=""}, operation (0:open)=T3."open or create") -> (refnum out=w264:refnum<file>, error out=w262:errorcluster)  [unwired: 3 in, 1 out]
        n160 = Set File Position(refnum=w264, from (0:start)=enum16{"start", "end", "current"}."end", error in=w262) -> (refnum out=w266:refnum<file>, error out=w265:errorcluster)  [unwired: 1 in]
        n161 = local read "Двиг част Hz"() -> (w243:string)
        n162 = local read "Двиг Ток А"() -> (w242:string)
        n163 = local read "T1"() -> (w250:string)
        n164 = local read "T2"() -> (w249:string)
        n165 = local read "T3"() -> (w248:string)
        n166 = local read "T4"() -> (w247:string)
        n167 = local read "T5"() -> (w246:string)
        n168 = local read "T6"() -> (w245:string)
        n169 = local read "T7"() -> (w244:string)
        n170 = Concatenate Strings(w252, w241, w250, w241, w249, w241, w248, w241, w247, w241, w246, w241, w245, w241, w244, w241, w243, w241, w242, w241, "\r") -> (w254:string)
        n171 = Write to Text File(file (use dialog)=w266, text=w254, error in=w265) -> (refnum out=w267:refnum<file>, error out=w268:errorcluster)  [unwired: 1 in, 1 out]
        n172 = Close File(refnum=w267, error in=w268) -> (error out=w269:errorcluster)  [unwired: 1 out]
        n173 = Unbundle(w269) -> ()  [unwired: 3 out]
        n174 = local read "Команда выход"() -> (w251:bool)
      }
      n175 = while {
        stop <- w58 stop-if-true
        # "Отображение времени на экране"
        n176 = Get Date/Time In Seconds() -> (seconds since 1Jan1904=w59:timestamp)
        n177 = Wait Until Next ms Multiple(millisecond multiple=u32 1000) -> ()  [unwired: 1 out]
        n178 = Format Date/Time String(time format string (%c)="%H:%M:%S", seconds (now)=w59) -> (date/time string=→"текущее время":string)  [unwired: 1 in]
        n179 = local read "Команда выход"() -> (w58:bool)
      }
      n180 = while {
        stop <- w310 stop-if-true
        # "Разбор и индикация входов и макро"
        # "Разбор и индикация входов и макро"
        n181 = Number To Decimal String(number="S1 v 2") -> (decimal integer string=→"Уч1 выд зад":string)  [unwired: 1 in]
        n182 = Number To Decimal String(number="S1 t 2") -> (decimal integer string=→"Уч1 Т зад":string)  [unwired: 1 in]
        n183 = Number To Boolean Array(number="X40-X77") -> (Boolean array=w352:bool[])
        n184 = Number To Boolean Array(number="X100-X137") -> (Boolean array=w334:bool[])
        n185 = Number To Decimal String(number="T2") -> (decimal integer string=→"T2":string)  [unwired: 1 in]
        n186 = Number To Decimal String(number="T4") -> (decimal integer string=→"T4":string)  [unwired: 1 in]
        n187 = Number To Decimal String(number="T1") -> (decimal integer string=→"T1":string)  [unwired: 1 in]
        n188 = Number To Decimal String(number="T3") -> (decimal integer string=→"T3":string)  [unwired: 1 in]
        n189 = Number To Decimal String(number="T5") -> (decimal integer string=→"T5":string)  [unwired: 1 in]
        n190 = Number To Decimal String(number="T7") -> (decimal integer string=→"T7":string)  [unwired: 1 in]
        n191 = Number To Decimal String(number="T6") -> (decimal integer string=→"T6":string)  [unwired: 1 in]
        n192 = Number To Decimal String(number="Cal v") -> (decimal integer string=→"Зак выд":string)  [unwired: 1 in]
        n193 = Wait Until Next ms Multiple(millisecond multiple=u32 1000) -> ()  [unwired: 1 out]
        n194 = Index Array(array=w352, index #1=7, index #2=8, index #3=9, index #4=10, index #5=16, index #6=17, index #7=18, index #8=0, index #9=0, index #10=0) -> (element #1=→"УПРАВЛЕНИЕ С PLC":bool, element #2=→"Авария привода":bool, element #3=→"Нагрев включен":bool, element #4=→"Готовность привода":bool, element #5=→"РАЗГРУЗКА":bool, element #6=→"ТОЧКА А":bool, element #7=→"ЗАЦЕП":bool)  [unwired: 3 out]
        n195 = Index Array(array=w334, index #1=0, index #2=1, index #3=4, index #4=5, index #5=8, index #6=10, index #7=11, index #8=16, index #9=17, index #10=18, index #11=19) -> (element #1=→"ПОД ОТКРЫТ":bool, element #2=→"ПОД ЗАКРЫТ":bool, element #3=→"Цепи вверху":bool, element #4=→"Цепи внизу":bool, element #5=→"Цепи среднее":bool, element #6=→"Домкрат вверху":bool, element #7=→"Домкрат внизу":bool, element #8=→"ВОДА":bool, element #9=→"ВОДА 2":bool, element #10=→"ВОДА 3":bool, element #11=→"ВОДА 4":bool)
        n196 = Number To Decimal String(number="Cal v 2") -> (decimal integer string=→"Зак зад":string)  [unwired: 1 in]
        n197 = Number To Decimal String(number="S2 t 2") -> (decimal integer string=→"Уч2 Тзад":string)  [unwired: 1 in]
        n198 = Number To Decimal String(number="S2v 2") -> (decimal integer string=→"Уч2 Выд зад":string)  [unwired: 1 in]
        n199 = Number To Decimal String(number="Hz") -> (decimal integer string=→"Двиг част Hz":string)  [unwired: 1 in]
        n200 = Number To Decimal String(number="A") -> (decimal integer string=→"Двиг Ток А":string)  [unwired: 1 in]
        n201 = Number To Decimal String(number="S1 v") -> (decimal integer string=→"Уч1 Выд":string)  [unwired: 1 in]
        n202 = Number To Decimal String(number="S1 t") -> (decimal integer string=→"Уч1 Т":string)  [unwired: 1 in]
        n203 = Number To Decimal String(number="S2v") -> (decimal integer string=→"Уч2 Выд":string)  [unwired: 1 in]
        n204 = Number To Decimal String(number="S2 t") -> (decimal integer string=→"Уч2 Т":string)  [unwired: 1 in]
        n205 = local read "Команда выход"() -> (w310:bool)
      }
    }
    frame #2 {
      # "Закрытие файла отчета"
      # "Закрытие файла отчета"
      n206 = local write "Команда выход"(FALSE ("Команда выход")) -> ()
    }
    frame #3 {
      # "Сохранение графика"
      # "Сохранение графика"
    }
    frame #4 {
      # "Закрытие программы"
      # "Закрытие программы"
      n207 = Quit LabVIEW() -> ()  [unwired: 1 in]
    }
  }
  n208 = case shown="True" FALSE {
    frame False {
    }
    frame True {
      n209 = call "Экран наладки.vi"() -> ()  [unwired: 12 in]
      n210 = call "NUMPAD1_9.vi"("МИНИМАЛЬНОЕ ЗНАЧЕНИЕ"=-1.0, "МАКСИМАЛЬНОЕ ЗНАЧЕНИЕ"=9999.0, "ДЛИННА СЛОВА"=i8 4, "ТЕКУЩЕЕ ЗНАЧЕНИЕ"="") -> ("НОВОЕ ЗНАЧЕНИЕ"=w360:string)  [unwired: 7 in]
      n211 = Decimal String To Number(string=w360) -> (number=w355:i32)  [unwired: 2 in, 1 out]
      n212 = DataSocket Write(8:errorcluster {"status"=FALSE, "code"=0, "source"=""} ("error in (no error)"), 9:100 ("ms timeout (0)"), 10:w355, 11:"opc://localhost/National Instruments.NIOPCServers/DL.DL260.v" ("connection in")) -> (0:w364:errorcluster)  [unwired: 2 out]
      n213 = Unbundle(w364) -> ()  [unwired: 3 out]
    }
  }
